vi "PCO_SetTimingStruct.vi"(8 "error in (no error)":errorcluster {"code" format="%x"}, 10 "strTiming":T1, 11 "ph":u64) -> (0 "error out":errorcluster {"code" format="%x"}, 2 "ErrorMessage":i32 format="%x", 3 "ph out":u64)   [LabVIEW 2019, in "SDK.lvlib" / "TimingControl.lvlib"]
doc: "<b>Description:</b>\nThis function does set the complete set of the timing settings. For the sake of clarity it is better to use the functions which change distinct parameter despite changing all settings at once.\nAn invalid value for one of the parameters will result in a failure response message.\nIf a single exposure/delay pair is to be set, the user must set all of the table members to zero except the first member 0. The table member 0 will hold the value for the single delay / exposure pair.\n\n<b>Supported camera type:</b>\nAll cameras\n\n<b>Descriptor dependency:</b>\nNone"
uses:
  TimingControl.lvlib
  Structures/Structures.lvlib
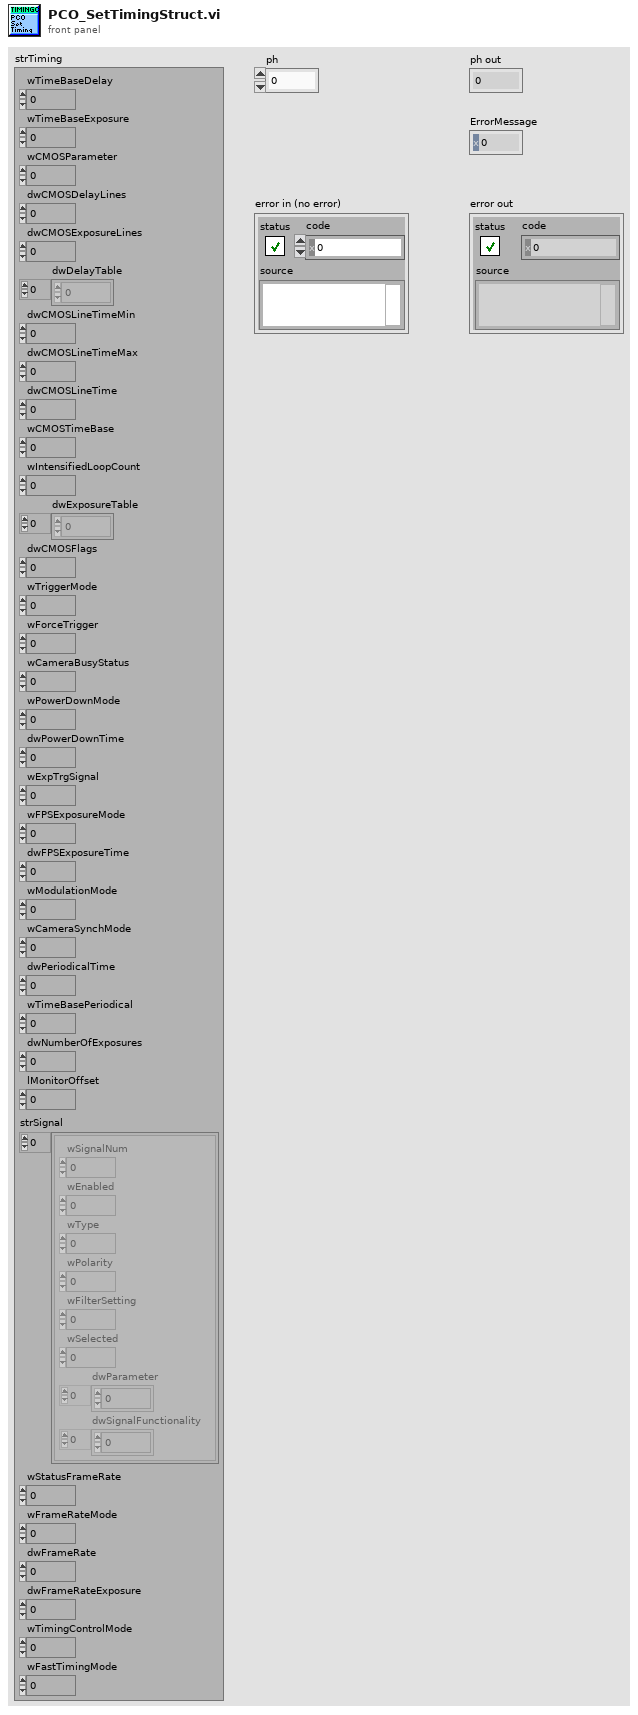
[diagram p1: front panel]
types:
  T1 = cluster{"wTimeBaseDelay":u16, "wTimeBaseExposure":u16, "wCMOSParameter":u16, "dwCMOSDelayLines":u32, "dwCMOSExposureLines":u32, "dwDelayTable":u32[], "dwCMOSLineTimeMin":u32, "dwCMOSLineTimeMax":u32, "dwCMOSLineTime":u32, "wCMOSTimeBase":u16, "wIntensifiedLoopCount":u16, "dwExposureTable":u32[], "dwCMOSFlags":u32, "wTriggerMode":u16, "wForceTrigger":u16, "wCameraBusyStatus":u16, "wPowerDownMode":u16, "dwPowerDownTime":u32, "wExpTrgSignal":u16, "wFPSExposureMode":u16, "dwFPSExposureTime":u32, "wModulationMode":u16, "wCameraSynchMode":u16, "dwPeriodicalTime":u32, "wTimeBasePeriodical":u16, "dwNumberOfExposures":u32, "lMonitorOffset":i32, "strSignal":cluster{"wSignalNum":u16, "wEnabled":u16, "wType":u16, "wPolarity":u16, "wFilterSetting":u16, "wSelected":u16, "dwParameter":u32[], "dwSignalFunctionality":u32[]}[], "wStatusFrameRate":u16, "wFrameRateMode":u16, "dwFrameRate":u32, "dwFrameRateExposure":u32, "wTimingControlMode":u16, "wFastTimingMode":u16}
  T2 = cluster{"wSignalNum":u16, "wEnabled":u16, "wType":u16, "wPolarity":u16, "wFilterSetting":u16, "wSelected":u16, "dwParameter":u32[], "dwSignalFunctionality":u32[]}[]
  T3 = cluster{"wSize":u16, "wSignalNum":u16, "wEnabled":u16, "wType":u16, "wPolarity":u16, "wFilterSetting":u16, "wSelected":u16, "ZZwReserved":u16, "dwParameter":cluster{u32, u32, u32, u32}, "dwSignalFunctionality":cluster{u32, u32, u32, u32}, "ZZdwReserved":cluster{u32, u32, u32}}
  T4 = cluster{"wSize":u16, "wSignalNum":u16, "wEnabled":u16, "wType":u16, "wPolarity":u16, "wFilterSetting":u16, "wSelected":u16, "ZZwReserved":u16, "dwParameter":cluster{u32, u32, u32, u32}, "dwSignalFunctionality":cluster{u32, u32, u32, u32}, "ZZdwReserved":cluster{u32, u32, u32}}[]
  T5 = cluster{"dwParameter[0]":u32, "dwParameter[1]":u32, "dwParameter[2]":u32, "dwParameter[3]":u32}
  T6 = cluster{"dwSignalFunctionality[0]":u32, "dwSignalFunctionality[1]":u32, "dwSignalFunctionality[2]":u32, "dwSignalFunctionality[3]":u32}
  T7 = cluster{"wSize":u16, "wTimeBaseDelay":u16, "wTimeBaseExposure":u16, "wCMOSParameter":u16, "dwCMOSDelayLines":u32, "dwCMOSExposureLines":u32, "dwDelayTable":cluster{u32, u32, u32, u32, u32, u32, u32, u32, u32, u32, u32, u32, u32, u32, u32, u32}, "ZZdwDummy1":cluster{"element":u32, "element 2":u32, "element 3":u32, "element 4":u32, "element 5":u32, "element 6":u32, "element 7":u32, "element 8":u32, "element 9":u32, "element 10":u32, "element 11":u32, "element 12":u32, "element 13":u32, "element 14":u32, "element 15":u32, "element 16":u32, "element 17":u32, "element 18":u32, "element 19":u32, "element 20":u32, "element 21":u32, "element 22":u32, "element 23":u32, "element 24":u32, "element 25":u32, "element 26":u32, "element 27":u32, "element 28":u32, "element 29":u32, "element 30":u32, "element 31":u32, "element 32":u32, "element 33":u32, "element 34":u32, "element 35":u32, "element 36":u32, "element 37":u32, "element 38":u32, "element 39":u32, "element 40":u32, "element 41":u32, "element 42":u32, "element 43":u32, "element 44":u32, "element 45":u32, "element 46":u32, "element 47":u32, "element 48":u32, "element 49":u32, "element 50":u32, "element 51":u32, "element 52":u32, "element 53":u32, "element 54":u32, "element 55":u32, "element 56":u32, "element 57":u32, "element 58":u32, "element 59":u32, "element 60":u32, "element 61":u32, "element 62":u32, "element 63":u32, "element 64":u32, "element 65":u32, "element 66":u32, "element 67":u32, "element 68":u32, "element 69":u32, "element 70":u32, "element 71":u32, "element 72":u32, "element 73":u32, "element 74":u32, "element 75":u32, "element 76":u32, "element 77":u32, "element 78":u32, "element 79":u32, "element 80":u32, "element 81":u32, "element 82":u32, "element 83":u32, "element 84":u32, "element 85":u32, "element 86":u32, "element 87":u32, "element 88":u32, "element 89":u32, "element 90":u32, "element 91":u32, "element 92":u32, "element 93":u32, "element 94":u32, "element 95":u32, "element 96":u32, "element 97":u32, "element 98":u32, "element 99":u32, "element 100":u32, "element 101":u32, "element 102":u32, "element 103":u32, "element 104":u32, "element 105":u32, "element 106":u32, "element 107":u32, "element 108":u32, "element 109":u32, "element 110":u32}, "dwCMOSLineTimeMin":u32, "dwCMOSLineTimeMax":u32, "dwCMOSLineTime":u32, "wCMOSTimeBase":u16, "wIntensifiedLoopCount":u16, "dwExposureTable":cluster{u32, u32, u32, u32, u32, u32, u32, u32, u32, u32, u32, u32, u32, u32, u32, u32}, "ZZdwDummy2":cluster{"element":u32, "element 2":u32, "element 3":u32, "element 4":u32, "element 5":u32, "element 6":u32, "element 7":u32, "element 8":u32, "element 9":u32, "element 10":u32, "element 11":u32, "element 12":u32, "element 13":u32, "element 14":u32, "element 15":u32, "element 16":u32, "element 17":u32, "element 18":u32, "element 19":u32, "element 20":u32, "element 21":u32, "element 22":u32, "element 23":u32, "element 24":u32, "element 25":u32, "element 26":u32, "element 27":u32, "element 28":u32, "element 29":u32, "element 30":u32, "element 31":u32, "element 32":u32, "element 33":u32, "element 34":u32, "element 35":u32, "element 36":u32, "element 37":u32, "element 38":u32, "element 39":u32, "element 40":u32, "element 41":u32, "element 42":u32, "element 43":u32, "element 44":u32, "element 45":u32, "element 46":u32, "element 47":u32, "element 48":u32, "element 49":u32, "element 50":u32, "element 51":u32, "element 52":u32, "element 53":u32, "element 54":u32, "element 55":u32, "element 56":u32, "element 57":u32, "element 58":u32, "element 59":u32, "element 60":u32, "element 61":u32, "element 62":u32, "element 63":u32, "element 64":u32, "element 65":u32, "element 66":u32, "element 67":u32, "element 68":u32, "element 69":u32, "element 70":u32, "element 71":u32, "element 72":u32, "element 73":u32, "element 74":u32, "element 75":u32, "element 76":u32, "element 77":u32, "element 78":u32, "element 79":u32, "element 80":u32, "element 81":u32, "element 82":u32, "element 83":u32, "element 84":u32, "element 85":u32, "element 86":u32, "element 87":u32, "element 88":u32, "element 89":u32, "element 90":u32, "element 91":u32, "element 92":u32, "element 93":u32, "element 94":u32, "element 95":u32, "element 96":u32, "element 97":u32, "element 98":u32, "element 99":u32, "element 100":u32, "element 101":u32, "element 102":u32, "element 103":u32, "element 104":u32, "element 105":u32, "element 106":u32, "element 107":u32, "element 108":u32, "element 109":u32, "element 110":u32}, "dwCMOSFlags":u32, "ZZdwDummy3":u32, "wTriggerMode":u16, "wForceTrigger":u16, "wCameraBusyStatus":u16, "wPowerDownMode":u16, "dwPowerDownTime":u32, "wExpTrgSignal":u16, "wFPSExposureMode":u16, "dwFPSExposureTime":u32, "wModulationMode":u16, "wCameraSynchMode":u16, "dwPeriodicalTime":u32, "wTimeBasePeriodical":u16, "ZZwDummy3":u16, "dwNumberOfExposures":u32, "lMonitorOffset":i32, "strSignal":cluster{"PCO_Signal_Raw":cluster{"wSize":u16, "wSignalNum":u16, "wEnabled":u16, "wType":u16, "wPolarity":u16, "wFilterSetting":u16, "wSelected":u16, "ZZwReserved":u16, "dwParameter":cluster{u32, u32, u32, u32}, "dwSignalFunctionality":cluster{u32, u32, u32, u32}, "ZZdwReserved":cluster{u32, u32, u32}}, "PCO_Signal_Raw":cluster{"wSize":u16, "wSignalNum":u16, "wEnabled":u16, "wType":u16, "wPolarity":u16, "wFilterSetting":u16, "wSelected":u16, "ZZwReserved":u16, "dwParameter":cluster{u32, u32, u32, u32}, "dwSignalFunctionality":cluster{u32, u32, u32, u32}, "ZZdwReserved":cluster{u32, u32, u32}}, "PCO_Signal_Raw":cluster{"wSize":u16, "wSignalNum":u16, "wEnabled":u16, "wType":u16, "wPolarity":u16, "wFilterSetting":u16, "wSelected":u16, "ZZwReserved":u16, "dwParameter":cluster{u32, u32, u32, u32}, "dwSignalFunctionality":cluster{u32, u32, u32, u32}, "ZZdwReserved":cluster{u32, u32, u32}}, "PCO_Signal_Raw":cluster{"wSize":u16, "wSignalNum":u16, "wEnabled":u16, "wType":u16, "wPolarity":u16, "wFilterSetting":u16, "wSelected":u16, "ZZwReserved":u16, "dwParameter":cluster{u32, u32, u32, u32}, "dwSignalFunctionality":cluster{u32, u32, u32, u32}, "ZZdwReserved":cluster{u32, u32, u32}}, "PCO_Signal_Raw":cluster{"wSize":u16, "wSignalNum":u16, "wEnabled":u16, "wType":u16, "wPolarity":u16, "wFilterSetting":u16, "wSelected":u16, "ZZwReserved":u16, "dwParameter":cluster{u32, u32, u32, u32}, "dwSignalFunctionality":cluster{u32, u32, u32, u32}, "ZZdwReserved":cluster{u32, u32, u32}}, "PCO_Signal_Raw":cluster{"wSize":u16, "wSignalNum":u16, "wEnabled":u16, "wType":u16, "wPolarity":u16, "wFilterSetting":u16, "wSelected":u16, "ZZwReserved":u16, "dwParameter":cluster{u32, u32, u32, u32}, "dwSignalFunctionality":cluster{u32, u32, u32, u32}, "ZZdwReserved":cluster{u32, u32, u32}}, "PCO_Signal_Raw":cluster{"wSize":u16, "wSignalNum":u16, "wEnabled":u16, "wType":u16, "wPolarity":u16, "wFilterSetting":u16, "wSelected":u16, "ZZwReserved":u16, "dwParameter":cluster{u32, u32, u32, u32}, "dwSignalFunctionality":cluster{u32, u32, u32, u32}, "ZZdwReserved":cluster{u32, u32, u32}}, "PCO_Signal_Raw":cluster{"wSize":u16, "wSignalNum":u16, "wEnabled":u16, "wType":u16, "wPolarity":u16, "wFilterSetting":u16, "wSelected":u16, "ZZwReserved":u16, "dwParameter":cluster{u32, u32, u32, u32}, "dwSignalFunctionality":cluster{u32, u32, u32, u32}, "ZZdwReserved":cluster{u32, u32, u32}}, "PCO_Signal_Raw":cluster{"wSize":u16, "wSignalNum":u16, "wEnabled":u16, "wType":u16, "wPolarity":u16, "wFilterSetting":u16, "wSelected":u16, "ZZwReserved":u16, "dwParameter":cluster{u32, u32, u32, u32}, "dwSignalFunctionality":cluster{u32, u32, u32, u32}, "ZZdwReserved":cluster{u32, u32, u32}}, "PCO_Signal_Raw":cluster{"wSize":u16, "wSignalNum":u16, "wEnabled":u16, "wType":u16, "wPolarity":u16, "wFilterSetting":u16, "wSelected":u16, "ZZwReserved":u16, "dwParameter":cluster{u32, u32, u32, u32}, "dwSignalFunctionality":cluster{u32, u32, u32, u32}, "ZZdwReserved":cluster{u32, u32, u32}}, "PCO_Signal_Raw":cluster{"wSize":u16, "wSignalNum":u16, "wEnabled":u16, "wType":u16, "wPolarity":u16, "wFilterSetting":u16, "wSelected":u16, "ZZwReserved":u16, "dwParameter":cluster{u32, u32, u32, u32}, "dwSignalFunctionality":cluster{u32, u32, u32, u32}, "ZZdwReserved":cluster{u32, u32, u32}}, "PCO_Signal_Raw":cluster{"wSize":u16, "wSignalNum":u16, "wEnabled":u16, "wType":u16, "wPolarity":u16, "wFilterSetting":u16, "wSelected":u16, "ZZwReserved":u16, "dwParameter":cluster{u32, u32, u32, u32}, "dwSignalFunctionality":cluster{u32, u32, u32, u32}, "ZZdwReserved":cluster{u32, u32, u32}}, "PCO_Signal_Raw":cluster{"wSize":u16, "wSignalNum":u16, "wEnabled":u16, "wType":u16, "wPolarity":u16, "wFilterSetting":u16, "wSelected":u16, "ZZwReserved":u16, "dwParameter":cluster{u32, u32, u32, u32}, "dwSignalFunctionality":cluster{u32, u32, u32, u32}, "ZZdwReserved":cluster{u32, u32, u32}}, "PCO_Signal_Raw":cluster{"wSize":u16, "wSignalNum":u16, "wEnabled":u16, "wType":u16, "wPolarity":u16, "wFilterSetting":u16, "wSelected":u16, "ZZwReserved":u16, "dwParameter":cluster{u32, u32, u32, u32}, "dwSignalFunctionality":cluster{u32, u32, u32, u32}, "ZZdwReserved":cluster{u32, u32, u32}}, "PCO_Signal_Raw":cluster{"wSize":u16, "wSignalNum":u16, "wEnabled":u16, "wType":u16, "wPolarity":u16, "wFilterSetting":u16, "wSelected":u16, "ZZwReserved":u16, "dwParameter":cluster{u32, u32, u32, u32}, "dwSignalFunctionality":cluster{u32, u32, u32, u32}, "ZZdwReserved":cluster{u32, u32, u32}}, "PCO_Signal_Raw":cluster{"wSize":u16, "wSignalNum":u16, "wEnabled":u16, "wType":u16, "wPolarity":u16, "wFilterSetting":u16, "wSelected":u16, "ZZwReserved":u16, "dwParameter":cluster{u32, u32, u32, u32}, "dwSignalFunctionality":cluster{u32, u32, u32, u32}, "ZZdwReserved":cluster{u32, u32, u32}}, "PCO_Signal_Raw":cluster{"wSize":u16, "wSignalNum":u16, "wEnabled":u16, "wType":u16, "wPolarity":u16, "wFilterSetting":u16, "wSelected":u16, "ZZwReserved":u16, "dwParameter":cluster{u32, u32, u32, u32}, "dwSignalFunctionality":cluster{u32, u32, u32, u32}, "ZZdwReserved":cluster{u32, u32, u32}}, "PCO_Signal_Raw":cluster{"wSize":u16, "wSignalNum":u16, "wEnabled":u16, "wType":u16, "wPolarity":u16, "wFilterSetting":u16, "wSelected":u16, "ZZwReserved":u16, "dwParameter":cluster{u32, u32, u32, u32}, "dwSignalFunctionality":cluster{u32, u32, u32, u32}, "ZZdwReserved":cluster{u32, u32, u32}}, "PCO_Signal_Raw":cluster{"wSize":u16, "wSignalNum":u16, "wEnabled":u16, "wType":u16, "wPolarity":u16, "wFilterSetting":u16, "wSelected":u16, "ZZwReserved":u16, "dwParameter":cluster{u32, u32, u32, u32}, "dwSignalFunctionality":cluster{u32, u32, u32, u32}, "ZZdwReserved":cluster{u32, u32, u32}}, "PCO_Signal_Raw":cluster{"wSize":u16, "wSignalNum":u16, "wEnabled":u16, "wType":u16, "wPolarity":u16, "wFilterSetting":u16, "wSelected":u16, "ZZwReserved":u16, "dwParameter":cluster{u32, u32, u32, u32}, "dwSignalFunctionality":cluster{u32, u32, u32, u32}, "ZZdwReserved":cluster{u32, u32, u32}}}, "wStatusFrameRate":u16, "wFrameRateMode":u16, "dwFrameRate":u32, "dwFrameRateExposure":u32, "wTimingControlMode":u16, "wFastTimingMode":u16, "ZZwDummy":cluster{"element":u16, "element 2":u16, "element 3":u16, "element 4":u16, "element 5":u16, "element 6":u16, "element 7":u16, "element 8":u16, "element 9":u16, "element 10":u16, "element 11":u16, "element 12":u16, "element 13":u16, "element 14":u16, "element 15":u16, "element 16":u16, "element 17":u16, "element 18":u16, "element 19":u16, "element 20":u16, "element 22":u16, "element 23":u16, "element 24":u16, "element 25":u16}}
  T8 = cluster{"element":u32, "element 2":u32, "element 3":u32, "element 4":u32, "element 5":u32, "element 6":u32, "element 7":u32, "element 8":u32, "element 9":u32, "element 10":u32, "element 11":u32, "element 12":u32, "element 13":u32, "element 14":u32, "element 15":u32, "element 16":u32, "element 17":u32, "element 18":u32, "element 19":u32, "element 20":u32, "element 21":u32, "element 22":u32, "element 23":u32, "element 24":u32, "element 25":u32, "element 26":u32, "element 27":u32, "element 28":u32, "element 29":u32, "element 30":u32, "element 31":u32, "element 32":u32, "element 33":u32, "element 34":u32, "element 35":u32, "element 36":u32, "element 37":u32, "element 38":u32, "element 39":u32, "element 40":u32, "element 41":u32, "element 42":u32, "element 43":u32, "element 44":u32, "element 45":u32, "element 46":u32, "element 47":u32, "element 48":u32, "element 49":u32, "element 50":u32, "element 51":u32, "element 52":u32, "element 53":u32, "element 54":u32, "element 55":u32, "element 56":u32, "element 57":u32, "element 58":u32, "element 59":u32, "element 60":u32, "element 61":u32, "element 62":u32, "element 63":u32, "element 64":u32, "element 65":u32, "element 66":u32, "element 67":u32, "element 68":u32, "element 69":u32, "element 70":u32, "element 71":u32, "element 72":u32, "element 73":u32, "element 74":u32, "element 75":u32, "element 76":u32, "element 77":u32, "element 78":u32, "element 79":u32, "element 80":u32, "element 81":u32, "element 82":u32, "element 83":u32, "element 84":u32, "element 85":u32, "element 86":u32, "element 87":u32, "element 88":u32, "element 89":u32, "element 90":u32, "element 91":u32, "element 92":u32, "element 93":u32, "element 94":u32, "element 95":u32, "element 96":u32, "element 97":u32, "element 98":u32, "element 99":u32, "element 100":u32, "element 101":u32, "element 102":u32, "element 103":u32, "element 104":u32, "element 105":u32, "element 106":u32, "element 107":u32, "element 108":u32, "element 109":u32, "element 110":u32}
  T9 = cluster{"element":u16, "element 2":u16, "element 3":u16, "element 4":u16, "element 5":u16, "element 6":u16, "element 7":u16, "element 8":u16, "element 9":u16, "element 10":u16, "element 11":u16, "element 12":u16, "element 13":u16, "element 14":u16, "element 15":u16, "element 16":u16, "element 17":u16, "element 18":u16, "element 19":u16, "element 20":u16, "element 22":u16, "element 23":u16, "element 24":u16, "element 25":u16}
  T10 = cluster{"dwDelayTable[0]":u32, "dwDelayTable[1]":u32, "dwDelayTable[2]":u32, "dwDelayTable[3]":u32, "dwDelayTable[4]":u32, "dwDelayTable[5]":u32, "dwDelayTable[6]":u32, "dwDelayTable[7]":u32, "dwDelayTable[8]":u32, "dwDelayTable[9]":u32, "dwDelayTable[10]":u32, "dwDelayTable[11]":u32, "dwDelayTable[12]":u32, "dwDelayTable[13]":u32, "dwDelayTable[14]":u32, "dwDelayTable[15]":u32}
  T11 = cluster{"dwExposureTable[0]":u32, "dwExposureTable[1]":u32, "dwExposureTable[2]":u32, "dwExposureTable[3]":u32, "dwExposureTable[4]":u32, "dwExposureTable[5]":u32, "dwExposureTable[6]":u32, "dwExposureTable[7]":u32, "dwExposureTable[8]":u32, "dwExposureTable[9]":u32, "dwExposureTable[10]":u32, "dwExposureTable[11]":u32, "dwExposureTable[12]":u32, "dwExposureTable[13]":u32, "dwExposureTable[14]":u32, "dwExposureTable[15]":u32}
  T12 = cluster{"[0]":cluster{"wSize":u16, "wSignalNum":u16, "wEnabled":u16, "wType":u16, "wPolarity":u16, "wFilterSetting":u16, "wSelected":u16, "ZZwReserved":u16, "dwParameter":cluster{u32, u32, u32, u32}, "dwSignalFunctionality":cluster{u32, u32, u32, u32}, "ZZdwReserved":cluster{u32, u32, u32}}, "[1]":cluster{"wSize":u16, "wSignalNum":u16, "wEnabled":u16, "wType":u16, "wPolarity":u16, "wFilterSetting":u16, "wSelected":u16, "ZZwReserved":u16, "dwParameter":cluster{u32, u32, u32, u32}, "dwSignalFunctionality":cluster{u32, u32, u32, u32}, "ZZdwReserved":cluster{u32, u32, u32}}, "[2]":cluster{"wSize":u16, "wSignalNum":u16, "wEnabled":u16, "wType":u16, "wPolarity":u16, "wFilterSetting":u16, "wSelected":u16, "ZZwReserved":u16, "dwParameter":cluster{u32, u32, u32, u32}, "dwSignalFunctionality":cluster{u32, u32, u32, u32}, "ZZdwReserved":cluster{u32, u32, u32}}, "[3]":cluster{"wSize":u16, "wSignalNum":u16, "wEnabled":u16, "wType":u16, "wPolarity":u16, "wFilterSetting":u16, "wSelected":u16, "ZZwReserved":u16, "dwParameter":cluster{u32, u32, u32, u32}, "dwSignalFunctionality":cluster{u32, u32, u32, u32}, "ZZdwReserved":cluster{u32, u32, u32}}, "[4]":cluster{"wSize":u16, "wSignalNum":u16, "wEnabled":u16, "wType":u16, "wPolarity":u16, "wFilterSetting":u16, "wSelected":u16, "ZZwReserved":u16, "dwParameter":cluster{u32, u32, u32, u32}, "dwSignalFunctionality":cluster{u32, u32, u32, u32}, "ZZdwReserved":cluster{u32, u32, u32}}, "[5]":cluster{"wSize":u16, "wSignalNum":u16, "wEnabled":u16, "wType":u16, "wPolarity":u16, "wFilterSetting":u16, "wSelected":u16, "ZZwReserved":u16, "dwParameter":cluster{u32, u32, u32, u32}, "dwSignalFunctionality":cluster{u32, u32, u32, u32}, "ZZdwReserved":cluster{u32, u32, u32}}, "[6]":cluster{"wSize":u16, "wSignalNum":u16, "wEnabled":u16, "wType":u16, "wPolarity":u16, "wFilterSetting":u16, "wSelected":u16, "ZZwReserved":u16, "dwParameter":cluster{u32, u32, u32, u32}, "dwSignalFunctionality":cluster{u32, u32, u32, u32}, "ZZdwReserved":cluster{u32, u32, u32}}, "[7]":cluster{"wSize":u16, "wSignalNum":u16, "wEnabled":u16, "wType":u16, "wPolarity":u16, "wFilterSetting":u16, "wSelected":u16, "ZZwReserved":u16, "dwParameter":cluster{u32, u32, u32, u32}, "dwSignalFunctionality":cluster{u32, u32, u32, u32}, "ZZdwReserved":cluster{u32, u32, u32}}, "[8]":cluster{"wSize":u16, "wSignalNum":u16, "wEnabled":u16, "wType":u16, "wPolarity":u16, "wFilterSetting":u16, "wSelected":u16, "ZZwReserved":u16, "dwParameter":cluster{u32, u32, u32, u32}, "dwSignalFunctionality":cluster{u32, u32, u32, u32}, "ZZdwReserved":cluster{u32, u32, u32}}, "[9]":cluster{"wSize":u16, "wSignalNum":u16, "wEnabled":u16, "wType":u16, "wPolarity":u16, "wFilterSetting":u16, "wSelected":u16, "ZZwReserved":u16, "dwParameter":cluster{u32, u32, u32, u32}, "dwSignalFunctionality":cluster{u32, u32, u32, u32}, "ZZdwReserved":cluster{u32, u32, u32}}, "[10]":cluster{"wSize":u16, "wSignalNum":u16, "wEnabled":u16, "wType":u16, "wPolarity":u16, "wFilterSetting":u16, "wSelected":u16, "ZZwReserved":u16, "dwParameter":cluster{u32, u32, u32, u32}, "dwSignalFunctionality":cluster{u32, u32, u32, u32}, "ZZdwReserved":cluster{u32, u32, u32}}, "[11]":cluster{"wSize":u16, "wSignalNum":u16, "wEnabled":u16, "wType":u16, "wPolarity":u16, "wFilterSetting":u16, "wSelected":u16, "ZZwReserved":u16, "dwParameter":cluster{u32, u32, u32, u32}, "dwSignalFunctionality":cluster{u32, u32, u32, u32}, "ZZdwReserved":cluster{u32, u32, u32}}, "[12]":cluster{"wSize":u16, "wSignalNum":u16, "wEnabled":u16, "wType":u16, "wPolarity":u16, "wFilterSetting":u16, "wSelected":u16, "ZZwReserved":u16, "dwParameter":cluster{u32, u32, u32, u32}, "dwSignalFunctionality":cluster{u32, u32, u32, u32}, "ZZdwReserved":cluster{u32, u32, u32}}, "[13]":cluster{"wSize":u16, "wSignalNum":u16, "wEnabled":u16, "wType":u16, "wPolarity":u16, "wFilterSetting":u16, "wSelected":u16, "ZZwReserved":u16, "dwParameter":cluster{u32, u32, u32, u32}, "dwSignalFunctionality":cluster{u32, u32, u32, u32}, "ZZdwReserved":cluster{u32, u32, u32}}, "[14]":cluster{"wSize":u16, "wSignalNum":u16, "wEnabled":u16, "wType":u16, "wPolarity":u16, "wFilterSetting":u16, "wSelected":u16, "ZZwReserved":u16, "dwParameter":cluster{u32, u32, u32, u32}, "dwSignalFunctionality":cluster{u32, u32, u32, u32}, "ZZdwReserved":cluster{u32, u32, u32}}, "[15]":cluster{"wSize":u16, "wSignalNum":u16, "wEnabled":u16, "wType":u16, "wPolarity":u16, "wFilterSetting":u16, "wSelected":u16, "ZZwReserved":u16, "dwParameter":cluster{u32, u32, u32, u32}, "dwSignalFunctionality":cluster{u32, u32, u32, u32}, "ZZdwReserved":cluster{u32, u32, u32}}, "[16]":cluster{"wSize":u16, "wSignalNum":u16, "wEnabled":u16, "wType":u16, "wPolarity":u16, "wFilterSetting":u16, "wSelected":u16, "ZZwReserved":u16, "dwParameter":cluster{u32, u32, u32, u32}, "dwSignalFunctionality":cluster{u32, u32, u32, u32}, "ZZdwReserved":cluster{u32, u32, u32}}, "[17]":cluster{"wSize":u16, "wSignalNum":u16, "wEnabled":u16, "wType":u16, "wPolarity":u16, "wFilterSetting":u16, "wSelected":u16, "ZZwReserved":u16, "dwParameter":cluster{u32, u32, u32, u32}, "dwSignalFunctionality":cluster{u32, u32, u32, u32}, "ZZdwReserved":cluster{u32, u32, u32}}, "[18]":cluster{"wSize":u16, "wSignalNum":u16, "wEnabled":u16, "wType":u16, "wPolarity":u16, "wFilterSetting":u16, "wSelected":u16, "ZZwReserved":u16, "dwParameter":cluster{u32, u32, u32, u32}, "dwSignalFunctionality":cluster{u32, u32, u32, u32}, "ZZdwReserved":cluster{u32, u32, u32}}, "[19]":cluster{"wSize":u16, "wSignalNum":u16, "wEnabled":u16, "wType":u16, "wPolarity":u16, "wFilterSetting":u16, "wSelected":u16, "ZZwReserved":u16, "dwParameter":cluster{u32, u32, u32, u32}, "dwSignalFunctionality":cluster{u32, u32, u32, u32}, "ZZdwReserved":cluster{u32, u32, u32}}}
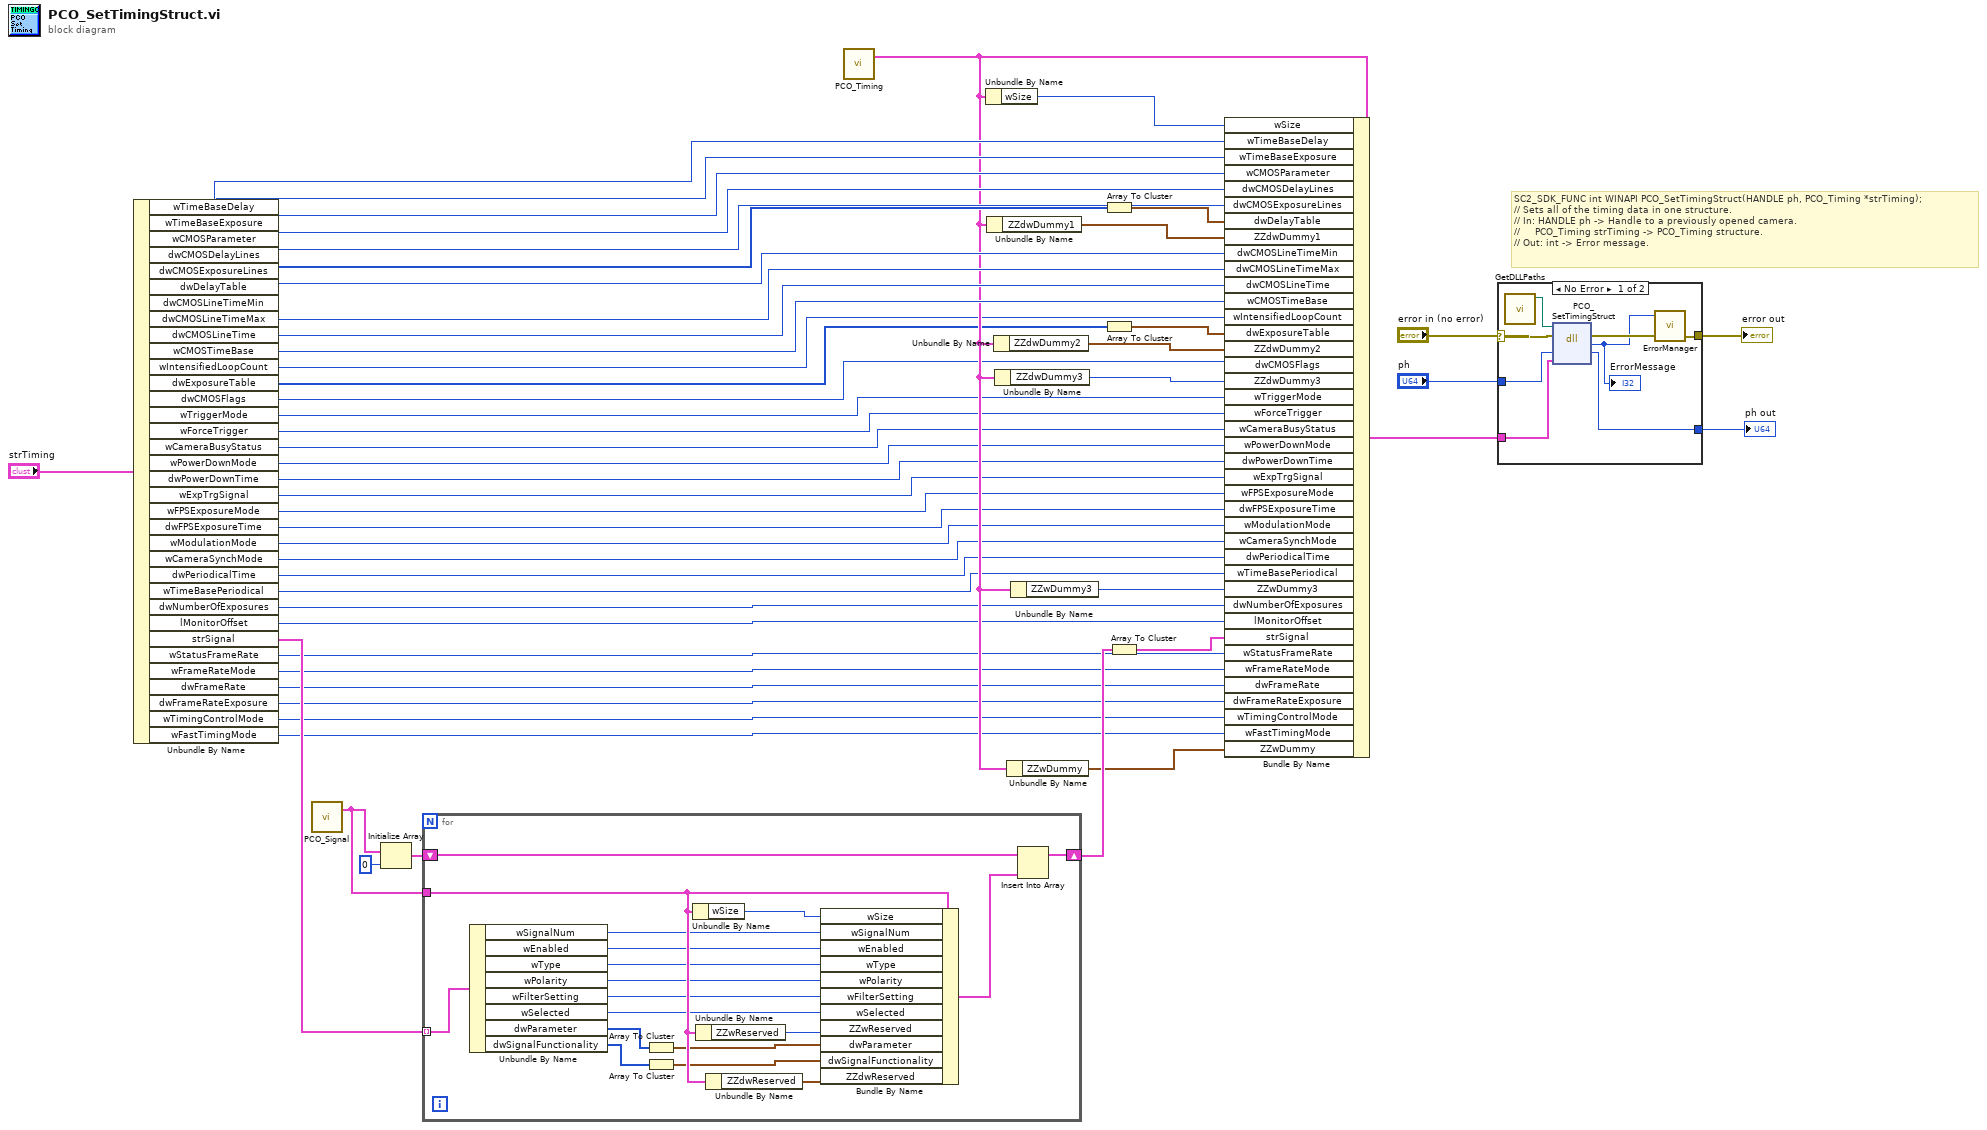
[diagram p0: block diagram]
diagram:
  # "SC2_SDK_FUNC int WINAPI PCO_SetTimingStruct(HANDLE ph, PCO_Timing *strTiming);\n// Sets all of the timing data in one structure.\n// In: HANDLE ph -> Handle to a previously opened camera.\n//     PCO_Timing strTiming -> PCO_Timing structure.\n// Out: int -> Error message."
  n1 = Unbundle By Name("strTiming") -> ("wTimeBaseDelay"=w43:u16, "wTimeBaseExposure"=w42:u16, "wCMOSParameter"=w41:u16, "dwCMOSDelayLines"=w40:u32, "dwCMOSExposureLines"=w39:u32, "dwDelayTable"=w46:u32[], "dwCMOSLineTimeMin"=w36:u32, "dwCMOSLineTimeMax"=w35:u32, "dwCMOSLineTime"=w34:u32, "wCMOSTimeBase"=w33:u16, "wIntensifiedLoopCount"=w27:u16, "dwExposureTable"=w26:u32[], "dwCMOSFlags"=w23:u32, "wTriggerMode"=w22:u16, "wForceTrigger"=w21:u16, "wCameraBusyStatus"=w20:u16, "wPowerDownMode"=w19:u16, "dwPowerDownTime"=w18:u32, "wExpTrgSignal"=w17:u16, "wFPSExposureMode"=w16:u16, "dwFPSExposureTime"=w15:u32, "wModulationMode"=w14:u16, "wCameraSynchMode"=w13:u16, "dwPeriodicalTime"=w12:u32, "wTimeBasePeriodical"=w11:u16, "dwNumberOfExposures"=w10:u32, "lMonitorOffset"=w9:i32, "strSignal"=w8:T2, "wStatusFrameRate"=w7:u16, "wFrameRateMode"=w6:u16, "dwFrameRate"=w5:u32, "dwFrameRateExposure"=w4:u32, "wTimingControlMode"=w3:u16, "wFastTimingMode"=w2:u16)
  n2 = call "PCO_Signal.vi"() -> ("PCO_Signal_Raw"=w48:T3)  [unwired: 4 in, 3 out]
  n3 = Initialize Array(w48, 0 ("dimension size")) -> (w49:T4)
  n4 = for {
    tunnel: w8 -> [w72] mode=indexing
    shift-right: [w57] -> w47
    shift-left: w49 -> [w55]
    tunnel: w48 -> [w69]
    n5 = Unbundle By Name(w72) -> ("wSignalNum"=w67:u16, "wEnabled"=w66:u16, "wType"=w65:u16, "wPolarity"=w64:u16, "wFilterSetting"=w63:u16, "wSelected"=w62:u16, "dwParameter"=w61:u32[], "dwSignalFunctionality"=w59:u32[])
    n6 = Array To Cluster(array=w61) -> (cluster=w60:T5)
    n7 = Array To Cluster(array=w59) -> (cluster=w58:T6)
    n8 = Unbundle By Name(w69) -> ("wSize"=w71:u16)
    n9 = Unbundle By Name(w69) -> ("ZZwReserved"=w70:u16)
    n10 = Unbundle By Name(w69) -> ("ZZdwReserved"=w68:cluster{u32, u32, u32})
    n11 = Bundle By Name(cluster=w69, "wSize"=w71, "wSignalNum"=w67, "wEnabled"=w66, "wType"=w65, "wPolarity"=w64, "wFilterSetting"=w63, "wSelected"=w62, "ZZwReserved"=w70, "dwParameter"=w60, "dwSignalFunctionality"=w58, "ZZdwReserved"=w68) -> (w56:T3)
    n12 = Insert Into Array(array=w55, new element=w56) -> (w57:T4)  [unwired: 1 in]
  }
  n13 = call "PCO_Timing.vi"() -> ("PCO_Timing_Raw"=w29:T7)  [unwired: 4 in, 3 out]
  n14 = Unbundle By Name(w29) -> ("wSize"=w44:u16)
  n15 = Unbundle By Name(w29) -> ("ZZdwDummy1"=w37:T8)
  n16 = Unbundle By Name(w29) -> ("ZZdwDummy2"=w25:T8)
  n17 = Unbundle By Name(w29) -> ("ZZdwDummy3"=w24:u32)
  n18 = Unbundle By Name(w29) -> ("ZZwDummy"=w30:T9)
  n19 = Unbundle By Name(w29) -> ("ZZwDummy3"=w31:u16)
  n20 = Array To Cluster(array=w46) -> (cluster=w38:T10)
  n21 = Array To Cluster(array=w26) -> (cluster=w32:T11)
  n22 = Array To Cluster(array=w47) -> (cluster=w28:T12)
  n23 = Bundle By Name(cluster=w29, "wSize"=w44, "wTimeBaseDelay"=w43, "wTimeBaseExposure"=w42, "wCMOSParameter"=w41, "dwCMOSDelayLines"=w40, "dwCMOSExposureLines"=w39, "dwDelayTable"=w38, "ZZdwDummy1"=w37, "dwCMOSLineTimeMin"=w36, "dwCMOSLineTimeMax"=w35, "dwCMOSLineTime"=w34, "wCMOSTimeBase"=w33, "wIntensifiedLoopCount"=w27, "dwExposureTable"=w32, "ZZdwDummy2"=w25, "dwCMOSFlags"=w23, "ZZdwDummy3"=w24, "wTriggerMode"=w22, "wForceTrigger"=w21, "wCameraBusyStatus"=w20, "wPowerDownMode"=w19, "dwPowerDownTime"=w18, "wExpTrgSignal"=w17, "wFPSExposureMode"=w16, "dwFPSExposureTime"=w15, "wModulationMode"=w14, "wCameraSynchMode"=w13, "dwPeriodicalTime"=w12, "wTimeBasePeriodical"=w11, "ZZwDummy3"=w31, "dwNumberOfExposures"=w10, "lMonitorOffset"=w9, "strSignal"=w28, "wStatusFrameRate"=w7, "wFrameRateMode"=w6, "dwFrameRate"=w5, "dwFrameRateExposure"=w4, "wTimingControlMode"=w3, "wFastTimingMode"=w2, "ZZwDummy"=w30) -> (w1:T7)
  n24 = case shown="No Error" "error in (no error)" {
    selector: "error in (no error)" -> [w77 w82]
    tunnel: "ph" -> [w80 w81]
    tunnel: [w79 w81] -> w53
    tunnel: w1 -> [w78 _]
    tunnel: [w75 w82] -> w52
    frame No Error {
      n25 = call "GetDLLPaths.vi"() -> ("SC2_Cam_Path"=w73:path)  [unwired: 8 in, 3 out]
      n26 = dll-call lib="?" fn="PCO_SetTimingStruct"(path in=w73, error in=w77, "ph"=w80, "strTiming"=w78) -> (error out=w76:errorcluster, "return type"=w74:i32, "ph"=w79:u64)  [unwired: 2 in, 1 out]
      "ErrorMessage" <- w74
      n27 = call "ErrorManager.vi"("error in (no error)"=w76, "error code"=w74) -> ("error out"=w75:errorcluster)  [unwired: 2 in, 1 out]
    }
    frame Error {
    }
  }
  "ph out" <- w53
  "error out" <- w52
